vi "GUI_laptop.vi"() -> ()   [LabVIEW 2019]
uses:
  <vilib>/Native 3D Graph/xcontrol/3DPC_SurfacePlot.xctl
  <vilib>/Platform/TimedLoop/XDataNode/timing_clust.ctl
  <vilib>/Platform/TimedLoop/XDataNode/nitl_modes.ctl
  <vilib>/Platform/TimedLoop/XDataNode/wakeup.ctl
  <vilib>/Instr/_visa.llb/VISA Configure Serial Port (Instr).vi
  <vilib>/Utility/file.llb/Write Delimited Spreadsheet (DBL).vi
  <vilib>/Analysis/BLAS.llb/dnrm2 - Vector 2-Norm (DBL).vi
  <vilib>/platform/TimedLoop/XDataNode/XDataNode.xnode
  <vilib>/Platform/TimedLoop/XDataNode/XDNodeRunTimeDep.lvlib
  <vilib>/Analysis/NI_AALBLAS.lvlib
panel:
  in  "Epsilon radius":dbl
  out "3D Graph":refnum<class "Base Datatype.lvclass">[](xcontrol)
  in  "Num of Points":i32
  in  "z bound":dbl
  in  "y bound":dbl
  in  "x bound":dbl
  in  "Stop":bool
  in  "Round Decimals":dbl format="%#_15g"
  in  "Save  Data":bool
  in  "Save Path":path
  in  "x speed":dbl
  in  "z speed":dbl
  in  "y speed":dbl
  out "error out":errorcluster
  in  "baud rate":u32=9600
  in  "VISA resource name":refnum<visa-resource-name>
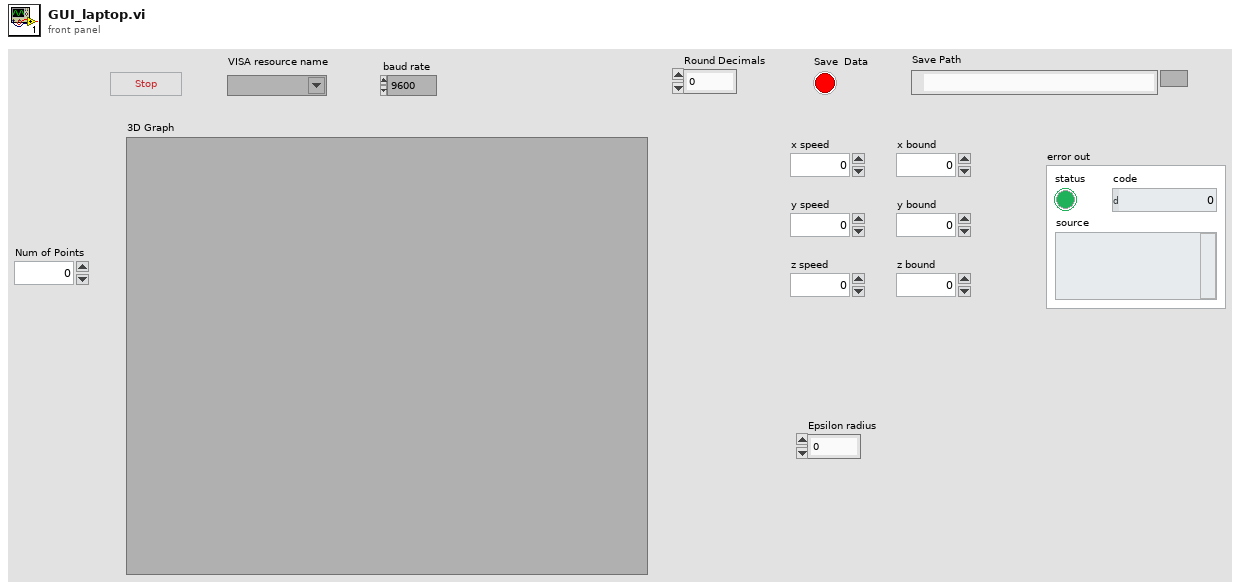
[diagram p1: front panel]
types:
  T1 = typedef "XDNodeRunTimeDep.lvlib/timing_clust.ctl" = cluster{"Expected End [f-1]":u64, "Actual End [f-1]":u64, "Finished Late? [f-1]":bool, "Expected End [i-1]":u64, "Actual End [i-1]":u64, "Finished Late? [i-1]":bool, "Expected Start [i]":u64, "Actual Start [i]":u64, "Expected Start [f]":u64, "Actual Start [f]":u64, "Source Name":string, "Structure Name":string, "Period":i64, "Deadline":i64, "Offset":i64, "Start":i64, "Priority":i32, "Timeout":i32, "Mode":T2, "Wakeup Reason":T3, "Error":errorcluster, "Source Type":string, "Secondary Source Type":string, "Global End Time":u64, "Global Start Time":u64, "Frame Duration":u64, "Iteration Duration":u64, "Assigned CPU":i32, "I/O Scan Engine Mode":u32}
  T2 = typedef "XDNodeRunTimeDep.lvlib/nitl_modes.ctl" = enum32{"No Change", "Process missed periods, maintain original phase", "Discard missed periods, maintain original phase", "Process missed periods, ignore original phase", "Discard missed periods, ignore original phase"}
  T3 = typedef "XDNodeRunTimeDep.lvlib/wakeup.ctl" = enum32{"Normal", "Aborted", "Asynchronous wakeup", "Timing source error", "Timed loop error", "Timeout"}
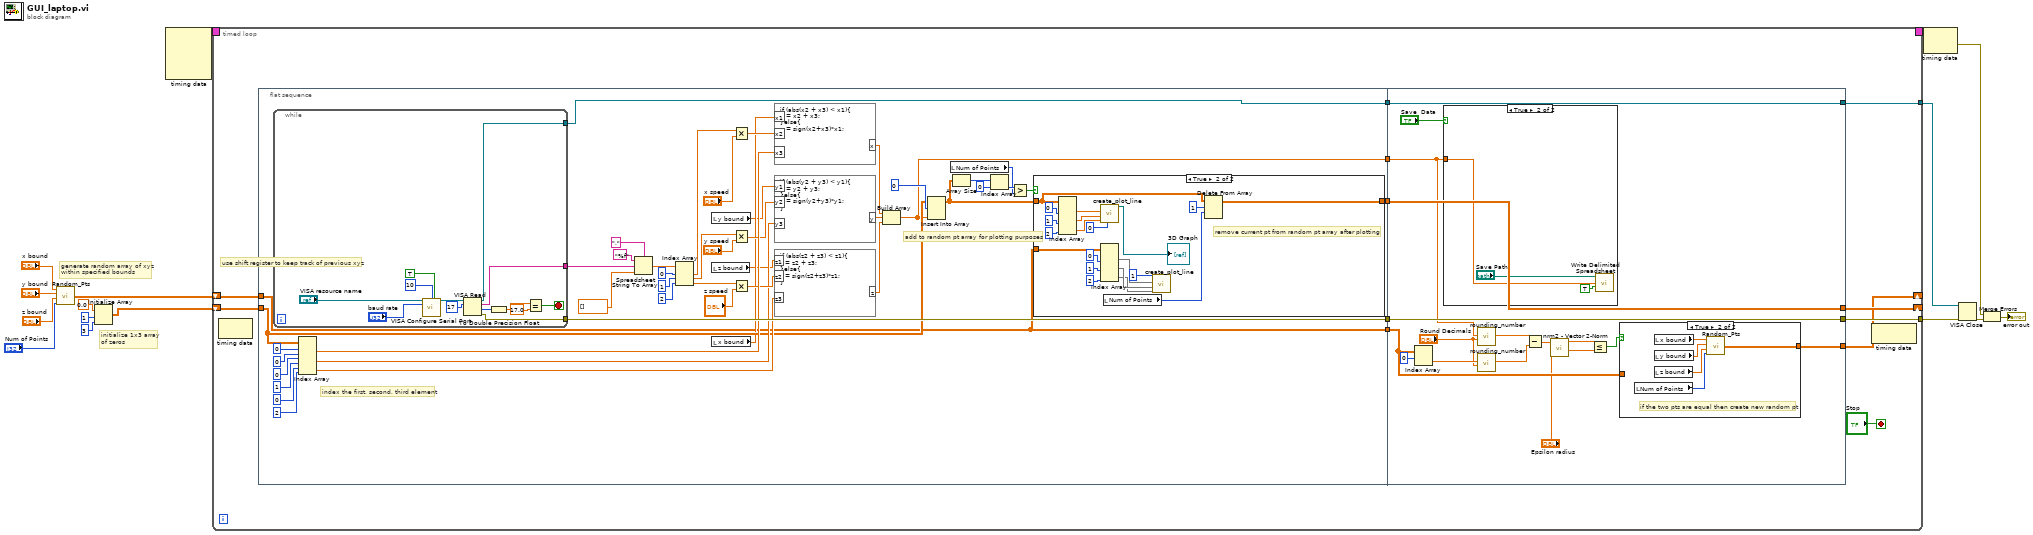
[diagram p0: block diagram]
diagram:
  # "generate random array of xyz\nwithin specified bounds"
  # "initialize 1x3 array \nof zeros"
  n1 = call "Random_Pts.vi"("Num of Points"="Num of Points", "z bound"="z bound", "y bound"="y bound", "x bound"="x bound") -> ("appended array"=w2:dbl[][])
  n2 = Initialize Array(0.0 ("element"), 1 ("dimension size"), 3 ("dimension size")) -> (w9:dbl[][])
  n3 = node-c288() -> (w16:T1)  [unwired: 4 in]
  n4 = timed-loop {
    tunnel: [w27] -> w11
    tunnel: [w26] -> w10
    shift-right: [w25] -> _
    shift-left: w9 -> [w24]
    timing: w16 -> [_]
    timing-out: [_] -> w15
    shift-right: [w17] -> _
    shift-left: w2 -> [w19]
    stop <- "Stop" stop-if-true
    # "use shift register to keep track of previous xyz"
    n5 = node-c288() -> ()  [unwired: 1 in, 1 out]
    n6 = flat-sequence {
      tunnel: w24 -> [w48]
      tunnel: [w34] -> w23
      tunnel: [w72] -> w22
      tunnel: [w36] -> w21
      tunnel: [w41] -> w20
      tunnel: w19 -> [w38]
      tunnel: [w38] -> w18
      tunnel: w23 -> [w125]
      tunnel: w22 -> [w124]
      tunnel: w21 -> [w123]
      tunnel: w20 -> [w117]
      tunnel: w18 -> [w119]
      tunnel: [w125] -> w27
      tunnel: [w124] -> w26
      tunnel: [w123] -> w25
      tunnel: [w118] -> w17
      frame #0 {
        # "add to random pt array for plotting purposes"
        # "index the first, second, third element"
        n7 = while {
          tunnel: [w108] -> w75
          tunnel: [w103] -> w72
          tunnel: [w97] -> w34
          stop <- w107 stop-if-true
          n8 = call-poly "VISA Configure Serial Port"("VISA resource name"="VISA resource name", "termination char\n(0xA = '\\n' = LF)"=u8 10 ("termination char\n(0xA = '\\n' = LF)"), "Enable Termination\nChar (T)"=TRUE ("Enable Termination\nChar (T)"), "baud rate (9600)"="baud rate") -> ("VISA resource name out"=w98:refnum<visa-resource-name>)  [unwired: 10 in, 1 out]
          n9 = VISA Read(VISA resource name=w98, byte count=u32 17) -> (VISA resource name out=w97:refnum<visa-resource-name>, read buffer=w108:string, return count=w105:u32, error out=w103:errorcluster)  [unwired: 1 in]
          n10 = To Double Precision Float(number=w105) -> (double precision float=w104:dbl)
          n11 = Equal?(x=w104, y=17.0 ("char count")) -> (x = y?=w107:bool)
        }
        n12 = Index Array(array=w48, index (row) #1=0 ("disabled index (row)"), index (col) #1=0 ("disabled index (col)"), index (row) #2=0 ("disabled index (row)"), index (col) #2=1 ("disabled index (col)"), index (row) #3=0 ("disabled index (row)"), index (col) #3=2 ("disabled index (col)")) -> (element #1=w62:dbl, element #2=w56:dbl, element #3=w59:dbl)
        n13 = Spreadsheet String To Array(delimiter (Tab)=",", format string="%f", spreadsheet string=w75, array type (2D Dbl)=dbl[] []) -> (array=w35:dbl[])
        n14 = Index Array(array=w35, index #1=0 ("index"), index #2=1 ("index"), index #3=2 ("index")) -> (element #1=w33:dbl, element #2=w32:dbl, element #3=w31:dbl)
        n15 = local read "y bound"() -> (w43:dbl)
        n16 = local read "z bound"() -> (w42:dbl)
        n17 = local read "x bound"() -> (w44:dbl)
        n18 = Multiply(x=w33, y="x speed") -> (x*y=w63:dbl)
        n19 = Multiply(x=w32, y="y speed") -> (x*y=w58:dbl)
        n20 = Multiply(x=w31, y="z speed") -> (x*y=w60:dbl)
        n21 = formula code="if (abs(x2 + x3) < x1){\nx = x2 + x3;\n}else{\nx = sign(x2+x3)*x1;\n}"("x1"=w44, "x2"=w63, "x3"=w62) -> ("x"=w52:dbl)
        n22 = formula code="if (abs(y2 + y3) < y1){\ny = y2 + y3;\n}else{\ny = sign(y2+y3)*y1;\n}"("y1"=w43, "y2"=w58, "y3"=w56) -> ("y"=w50:dbl)
        n23 = formula code="if (abs(z2 + z3) < z1){\nz = z2 + z3;\n}else{\nz = sign(z2+z3)*z1;\n}"("z1"=w42, "z2"=w60, "z3"=w59) -> ("z"=w51:dbl)
        n24 = Build Array(w52, w50, w51) -> (w41:dbl[])
        n25 = Insert Into Array(array=w48, index (row)=0, new element=w41) -> (w39:dbl[][])  [unwired: 1 in]
        n26 = local read "Num of Points"() -> (w40:i32)
        n27 = Array Size(array=w39) -> (size(s)=w49:i32[])
        n28 = Index Array(array=w49, index=0) -> (element=w53:i32)
        n29 = Greater?(x=w53, y=w40) -> (0:w37:bool)
        n30 = case shown="True" w37 {
          tunnel: w39 -> [w76 w92]
          tunnel: [w76 w91] -> w36
          tunnel: w38 -> [_ w90]
          frame False {
          }
          frame True {
            # "remove current pt from random pt array after plotting"
            n31 = Index Array(array=w92, index (col) #1=0 ("disabled index (col)"), index (col) #2=1 ("index (col)"), index (col) #3=2 ("index (col)")) -> (element #1=w83:dbl[], element #2=w82:dbl[], element #3=w81:dbl[])  [unwired: 3 in]
            n32 = call <vilib>:"create_plot_line.vi"("plot ID"=0, "z vector"=w81, "y vector"=w82, "x vector"=w83) -> ("plots out"=→"3D Graph":refnum<class "Base Datatype.lvclass">[])  [unwired: 1 in, 6 out]
            n33 = Index Array(array=w90, index (col) #1=0 ("disabled index (col)"), index (col) #2=1 ("index (col)"), index (col) #3=2 ("index (col)")) -> (element #1=w80:dbl[], element #2=w79:dbl[], element #3=w78:dbl[])  [unwired: 3 in]
            n34 = local read "Num of Points"() -> (w86:i32)
            n35 = call <vilib>:"create_plot_line.vi"("plot ID"=1, "z vector"=w78, "y vector"=w79, "x vector"=w80) -> ()  [unwired: 1 in, 7 out]
            n36 = Delete From Array(array=w92, length=1, index (row)=w86) -> (array with subset deleted=w91:dbl[][])  [unwired: 1 in, 1 out]
          }
        }
      }
      frame #1 {
        n37 = Index Array(array=w119, index (row)=0) -> (element=w121:dbl[])  [unwired: 1 in]
        n38 = case shown="True" "Save  Data" {
          tunnel: w117 -> [_ w126]
          frame False {
          }
          frame True {
            n39 = call-poly <vilib>:"Write Delimited Spreadsheet.vi"("file path (dialog if empty)"="Save Path", "1D data"=w126, "append to file? (new file:F)"=TRUE) -> ()  [unwired: 11 in, 2 out]
          }
        }
        n40 = call "rounding_number.vi"("power of ten"="Round Decimals", "Array"=w121) -> ("rounded"=w115:dbl[])  [unwired: 9 in]
        n41 = call "rounding_number.vi"("power of ten"="Round Decimals", "Array"=w117) -> ("rounded"=w114:dbl[])  [unwired: 9 in]
        n42 = Subtract(x=w114, y=w115) -> (x-y=w113:dbl[])
        n43 = call-poly <vilib>:"nrm2 - Vector 2-Norm.vi"("x"=w113) -> ("dnrm2"=w111:dbl)  [unwired: 9 in, 1 out]
        n44 = Less Or Equal?(x=w111, y="Epsilon radius") -> (x <= y?=w112:bool)
        n45 = case shown="True" w112 {
          tunnel: w119 -> [w129 _]
          tunnel: [w129 w130] -> w118
          frame False {
          }
          frame True {
            # "if the two pts are equal then create new random pt"
            n46 = local read "Num of Points"() -> (w131:i32)
            n47 = local read "x bound"() -> (w134:dbl)
            n48 = local read "y bound"() -> (w133:dbl)
            n49 = local read "z bound"() -> (w132:dbl)
            n50 = call "Random_Pts.vi"("Num of Points"=w131, "z bound"=w132, "y bound"=w133, "x bound"=w134) -> ("appended array"=w130:dbl[][])
          }
        }
      }
    }
    n51 = node-c288() -> ()  [unwired: 1 in, 1 out]
  }
  n52 = node-c288(w15) -> (w8:errorcluster)
  n53 = VISA Close(VISA resource name=w11, error in (no error)=w10) -> (error out=w7:errorcluster)
  n54 = Merge Errors(w8, w7) -> (→"error out":errorcluster)
